vi "Read_write.vi"(0 "Command":enum16{"SET", "DIS"}(ring), 1 "Function":T1(ring), 2 "Argument":string, 3 "error in (no error)":errorcluster, 4 "GPIB address":string) -> (5 "Message received":string, 6 "error out":errorcluster)   [LabVIEW 2010]
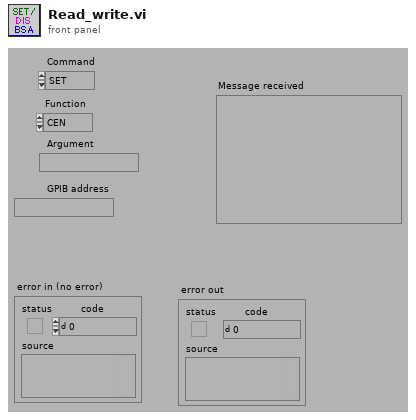
[diagram p1: front panel]
types:
  T1 = enum16{"CEN", "SPA", "SIG", "PED", "HIG", "REC", "MOD", "CAL", "WHO", "LOC", "REM"}
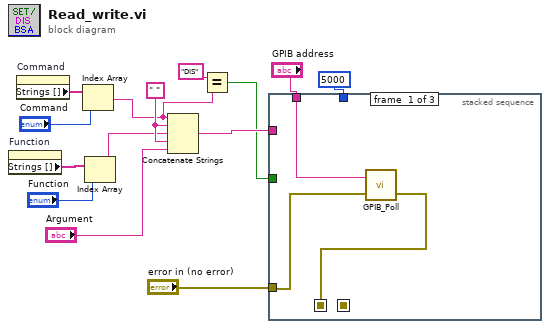
[diagram p0: block diagram]
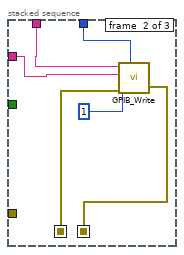
[diagram p2: hidden frame]
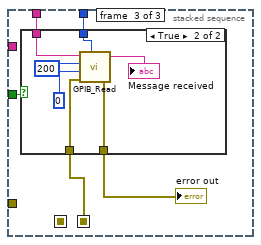
[diagram p3: hidden frame]
diagram:
  w9 = " "
  n1 = property on="Function" class="Enum (strict)"() -> ("Strings []"=w11:string[])  [unwired: 2 in, 2 out]
  n2 = property on="Command" class="Enum (strict)"() -> ("Strings []"=w13:string[])  [unwired: 2 in, 2 out]
  n3 = Index Array(array=w13, index="Command") -> (element=w4:string)
  n4 = Index Array(array=w11, index="Function") -> (element=w8:string)
  n5 = Concatenate Strings(w4, w9, w8, w9, "Argument") -> (w6:string)
  n6 = Equal?(x="DIS", y=w4) -> (x = y?=w3:bool)
  n7 = stacked-sequence {
    seq-local: [_ w19 _] -> [_ _ w25]
    seq-local: [w15 _ _] -> [_ w18 _]
    tunnel: "GPIB address" -> [w17 w23 w28]
    tunnel: 5000 -> [_ w21 w27]
    tunnel: w6 -> [_ w20 _]
    tunnel: w3 -> [_ _ w26]
    tunnel: "error in (no error)" -> [w16 _ _]
    frame #0 {
      n8 = call "GPIB_Poll.vi"("error in"=w16, "address string"=w17) -> ("error out"=w15:errorcluster)  [unwired: 1 out]
    }
    frame #1 {
      n9 = call "GPIB_Write.vi"("address string"=w23, "data In"=w20, "mode (0)"=i16 1, "error in"=w18, "timeout ms (488.2 global)"=w21) -> ("error out"=w19:errorcluster)  [unwired: 1 out]
    }
    frame #2 {
      n10 = case shown="True" w26 {
        tunnel: w27 -> [_ w34]
        tunnel: w28 -> [_ w35]
        tunnel: w25 -> [w29 w31]
        tunnel: [w29 w30] -> w24
        frame False {
        }
        frame True {
          n11 = call "GPIB_Read.vi"("address string"=w35, "byte count"=200, "mode (0)"=i16 0, "error in"=w31, "timeout ms (488.2 global)"=w34) -> ("data Out"=→"Message received":string, "error out"=w30:errorcluster)  [unwired: 1 out]
        }
      }
      "error out" <- w24
    }
  }
